vi "Initiate Colliders.vi"(2 "Simulation Objects in":refnum<class "SimulationObject.lvclass">[](array[class]), 3 "PhysicsSystem in":refnum<class "PhysicsSystem.lvclass">) -> (0 "Simulation Object out":refnum<class "SimulationObject.lvclass">[](array[class]), 1 "PhysicsSystem out":refnum<class "PhysicsSystem.lvclass">)   [LabVIEW 2022 SP3, in "PhysicsSystem.lvclass"]
uses:
  PhysicsSystem.lvclass
  Objects/SimulationObject/SimulationObject.lvclass
  PhysicsSystem.lvclass/PhysicsSystem.ctl
  Objects/SimulationObject/SimulationObject.lvclass/SimulationObject.ctl
  Objects/Collisions/Collider/Collider.lvclass/Collider.ctl
  Objects/Collisions/CollisionGrid/CollisionGrid.lvclass
  Objects/Collisions/Collider/Collider.lvclass
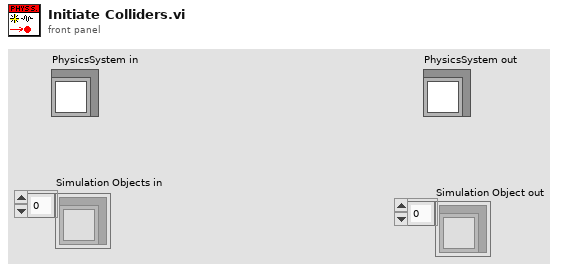
[diagram p1: front panel]
types:
  T1 = cluster{"x shift":i16, "y shift":i16, "x cells":i16, "y cells":i16}
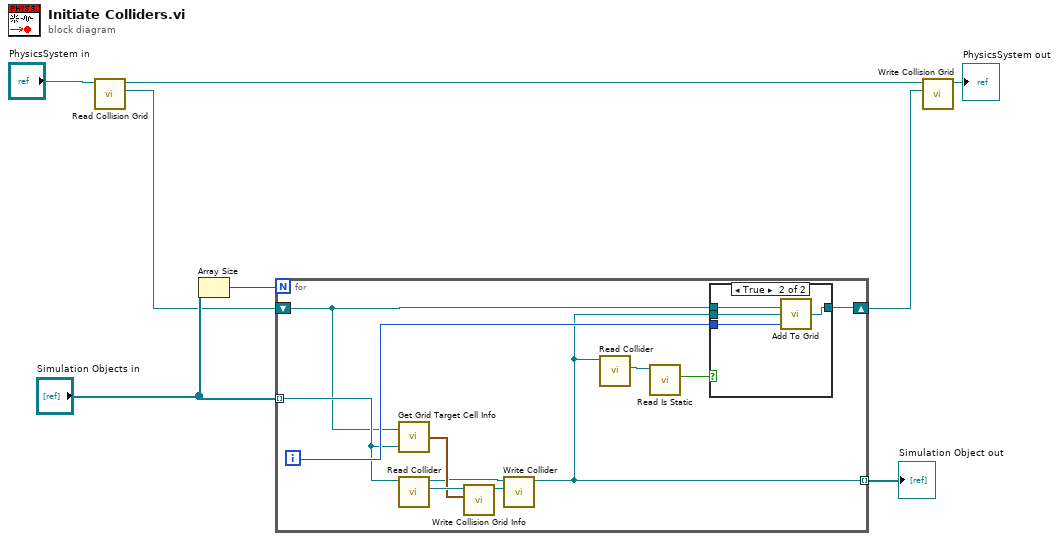
[diagram p0: block diagram]
diagram:
  n1 = call "Read Collision Grid.vi"("PhysicsSystem in"="PhysicsSystem in") -> ("Collision Grid out"=w6:refnum<class "CollisionGrid.lvclass">, "PhysicsSystem out"=w4:refnum<class "PhysicsSystem.lvclass">)  [unwired: 8 in, 1 out]
  n2 = Array Size(array="Simulation Objects in") -> (size(s)=w8:i32)
  n3 = for {
    N: w8 -> [_]
    tunnel: "Simulation Objects in" -> [w15] mode=indexing
    shift-right: [w19] -> w3
    shift-left: w6 -> [w14]
    tunnel: [w9] -> w1 mode=indexing
    i -> [w18]
    n4 = call "Get Grid Target Cell Info.vi"("Simulation Object in"=w15, "Collision Grid in"=w14) -> ("info"=w12:T1)
    n5 = call "Read Collider.vi"("SimulationObject in"=w15) -> ("Collider out"=w13:refnum<class "Collider.lvclass">, "SimulationObject out"=w11:refnum<class "SimulationObject.lvclass">)  [unwired: 8 in, 1 out]
    n6 = call "Write Collision Grid Info.vi"("Collision Grid Info"=w12, "Collider in"=w13) -> ("Collider out"=w10:refnum<class "Collider.lvclass">)  [unwired: 8 in, 1 out]
    n7 = call "Write Collider.vi"("Collider in"=w10, "SimulationObject in"=w11) -> ("SimulationObject out"=w9:refnum<class "SimulationObject.lvclass">)  [unwired: 8 in, 1 out]
    n8 = call "Read Collider.vi"("SimulationObject in"=w9) -> ("Collider out"=w17:refnum<class "Collider.lvclass">)  [unwired: 8 in, 2 out]
    n9 = call "Read Is Static.vi"("Collider in"=w17) -> ("Is Static"=w16:bool)  [unwired: 8 in, 2 out]
    n10 = case shown="True" w16 {
      tunnel: w14 -> [w20 w24]
      tunnel: [w20 w23] -> w19
      tunnel: w18 -> [_ w22]
      tunnel: w9 -> [_ w21]
      frame False {
      }
      frame True {
        n11 = call "Add To Grid.vi"("Object Index in"=w22, "Simulation Object in"=w21, "Collision Grid in"=w24) -> ("Collision Grid out"=w23:refnum<class "CollisionGrid.lvclass">)
      }
    }
  }
  "Simulation Object out" <- w1
  n12 = call "Write Collision Grid.vi"("CollisionGrid.lvclass"=w3, "PhysicsSystem in"=w4) -> ("PhysicsSystem out"=→"PhysicsSystem out":refnum<class "PhysicsSystem.lvclass">)  [unwired: 8 in, 1 out]
